vi "Get Team.vi"(8 "error in (no error)":errorcluster, 11 "Team Config Panel in":refnum<class "Team Config Panel.lvclass">) -> (0 "error out":errorcluster, 2 "Team":refnum<class "Team.lvclass">, 3 "Team Config Panel out":refnum<class "Team Config Panel.lvclass">)   [LabVIEW 2020, in "SB App.lvlib" / "Team Config Panel.lvclass"]
uses:
  Team Config Panel.lvclass
  SquareBattle/Team/Team.lvclass
  Team Config Panel.lvclass/Team Config Panel.ctl
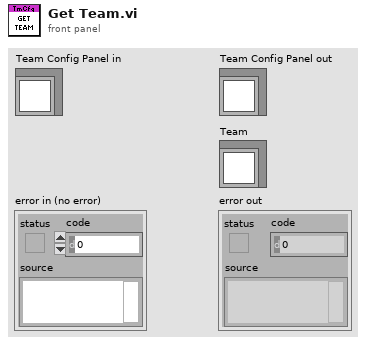
[diagram p1: front panel]
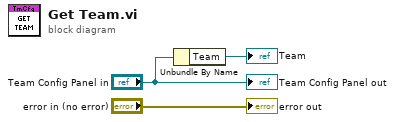
[diagram p0: block diagram]
diagram:
  n1 = Unbundle By Name("Team Config Panel in") -> ("Team"=→"Team":refnum<class "Team.lvclass">)
  "error out" <- "error in (no error)"
  "Team Config Panel out" <- "Team Config Panel in"
